vi "get_ecrh_duration.vi"(11 "default":dbl=40.0 format="%#_13g") -> (0 "HTTP status":i32, 1 "ecrh duration":dbl, 2 "time needed to find ECRH duration":i64, 3 "No. Trys":i32, 4 "date/time string":string, 5 "progId":dbl, 6 "last trigger time by codac":i64, 7 "Sucessfull HTTP return?":bool)   [LabVIEW 2014]
uses:
  <vilib>/regexp/Match Regular Expression.xnode
  <vilib>/httpClient/LabVIEWHTTPClient.lvlib
  <vilib>/LVH/i3 JSON/i3-json.lvlib
panel:
  out "is fine?":bool
  out "string length":i32
  out "whole match":string
  out "ECRH substring":string
  out "logbook body":string
  out "after match":string
  out "No. of Trys x > y?":bool
  out "loop status":bool
  out "Tick after":u32 caption="tick after"
  out "tick before":u32
  out "logbook header":string
  out "value":dbl[](array[numeric])
  out "JSON Tree":variant
  out "body":string
  out "headers":string
  out "concatenated string":string
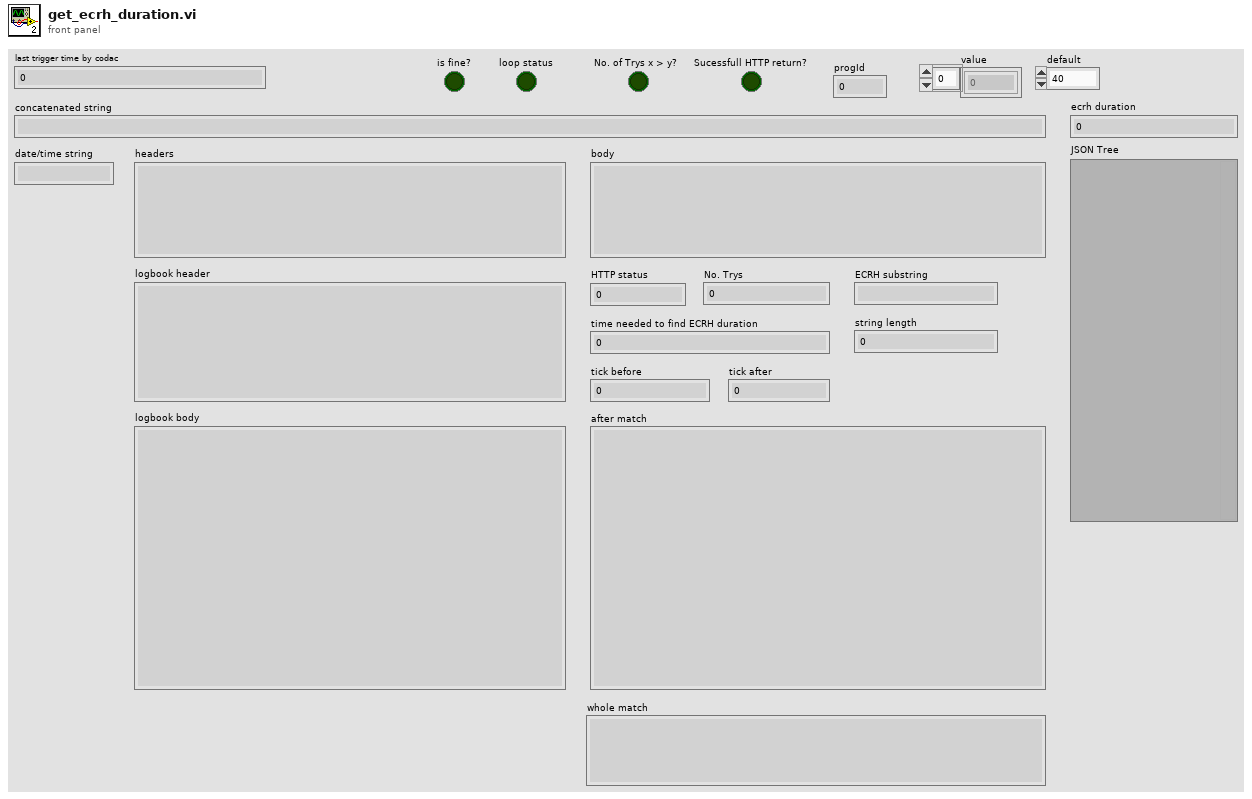
[diagram p1: front panel]
types:
  T1 = typedef "LabVIEWHTTPClient.lvlib/ClientHandle.ctl" = refnum<k1>
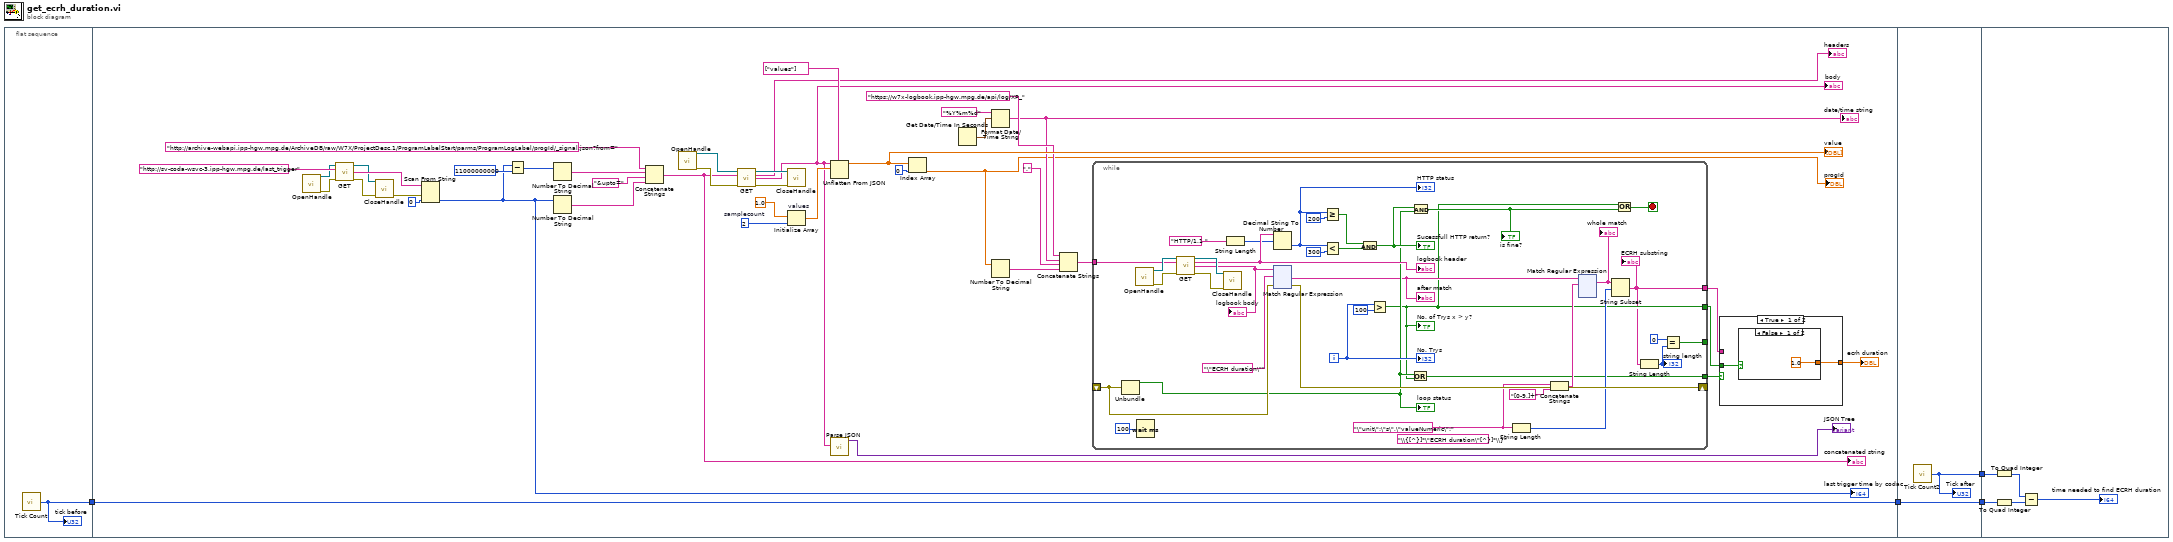
[diagram p0: block diagram]
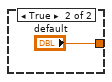
[diagram p2: hidden frame]
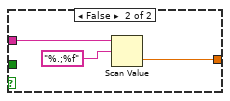
[diagram p3: hidden frame]
diagram:
  n1 = flat-sequence {
    tunnel: [w5] -> w3
    tunnel: [w9] -> w4
    tunnel: w3 -> [w9]
    tunnel: w4 -> [w320]
    tunnel: [w320] -> w2
    tunnel: [w319] -> w1
    tunnel: w2 -> [w324]
    tunnel: w1 -> [w323]
    frame #0 {
      n2 = call "Tick Count"() -> ("Tick Count(mSec)"=w5:u32)
      "tick before" <- w5
    }
    frame #1 {
      w24 = 2  # samplecount
      n3 = call <vilib>:"OpenHandle.vi"() -> ("client handle out"=w43:T1, "error out"=w46:errorcluster)  [unwired: 14 in]
      n4 = call <vilib>:"GET.vi"("client handle"=w43, "url"="http://sv-coda-wsvc-3.ipp-hgw.mpg.de/last_trigger", "error in (no error)"=w46) -> ("client handle out"=w42:T1, "body"=w45:string, "error out"=w41:errorcluster)  [unwired: 9 in, 1 out]
      n5 = call <vilib>:"CloseHandle.vi"("client handle"=w42, "error in (no error)"=w41) -> ("error out"=w40:errorcluster)  [unwired: 13 in]
      n6 = Scan From String(input string=w45, error in=w40, default 1=i64 0 ("default (0 I32)")) -> (output 1=w25:i64)  [unwired: 2 in, 3 out]
      "last trigger time by codac" <- w25
      n7 = Subtract(x=w25, y=i64 11000000000) -> (x-y=w35:i64)
      n8 = Number To Decimal String(number=w35) -> (decimal integer string=w34:string)  [unwired: 1 in]
      n9 = Number To Decimal String(number=w25) -> (decimal integer string=w32:string)  [unwired: 1 in]
      n10 = Concatenate Strings("http://archive-webapi.ipp-hgw.mpg.de/ArchiveDB/raw/W7X/ProjectDesc.1/ProgramLabelStart/parms/ProgramLogLabel/progId/_signal.json?from=", w34, "&upto=", w32) -> (w29:string)
      "concatenated string" <- w29
      n11 = call <vilib>:"OpenHandle.vi"() -> ("client handle out"=w28:T1, "error out"=w31:errorcluster)  [unwired: 14 in]
      n12 = call <vilib>:"GET.vi"("client handle"=w28, "url"=w29, "error in (no error)"=w31) -> ("client handle out"=w27:T1, "headers"=→"headers":string, "body"=w13:string, "error out"=w30:errorcluster)  [unwired: 9 in]
      "body" <- w13
      n13 = call <vilib>:"CloseHandle.vi"("client handle"=w27, "error in (no error)"=w30) -> ()  [unwired: 13 in, 1 out]
      n14 = Initialize Array "values"(1.0 ("element"), w24) -> (w22:dbl[])
      n15 = Unflatten From JSON(path=string[] ["values"], JSON string=w13, type and defaults=w22) -> (value=w21:dbl[])  [unwired: 4 in, 1 out]
      "value" <- w21
      n16 = call <vilib>:"Parse JSON.vi"("JSON String"=w13) -> ("JSON Tree"=→"JSON Tree":variant)  [unwired: 7 in, 3 out]
      n17 = Index Array(array=w21, index=0) -> (element=w16:dbl)
      "progId" <- w16
      n18 = Get Date/Time In Seconds() -> (seconds since 1Jan1904=w39:timestamp)
      n19 = Format Date/Time String(time format string (%c)="%Y%m%d", seconds (now)=w39) -> (date/time string=w18:string)  [unwired: 1 in]
      "date/time string" <- w18
      n20 = Number To Decimal String(number=w16) -> (decimal integer string=w15:string)  [unwired: 1 in]
      n21 = Concatenate Strings("https://w7x-logbook.ipp-hgw.mpg.de/api/log/XP_", w18, "." ("string"), w15) -> (w14:string)
      n22 = while {
        tunnel: w14 -> [w86]
        tunnel: [w60] -> w6
        shift-right: [w70] -> _
        shift-left: _ -> [w69]
        tunnel: [w59] -> w8
        tunnel: [w61] -> w7
        tunnel: [w56] -> _
        i -> [w76]
        stop <- w72 stop-if-true
        (unwired) "\\{[^}]*\"ECRH duration\"[^}]*\\}" ("regular expression")
        w55 = "\"unit\":\"s\",\"valueNumeric\":"
        n23 = Unbundle(w69) -> ("status"=w68:bool)  [unwired: 2 out]
        "loop status" <- w68
        n24 = call <vilib>:"OpenHandle.vi"() -> ("client handle out"=w88:T1, "error out"=w90:errorcluster)  [unwired: 14 in]
        n25 = Wait (ms)(milliseconds to wait=u32 100) -> ()  [unwired: 1 out]
        n26 = call <vilib>:"GET.vi"("client handle"=w88, "url"=w86, "error in (no error)"=w90) -> ("client handle out"=w87:T1, "headers"=w81:string, "body"=w74:string, "error out"=w89:errorcluster)  [unwired: 9 in]
        "logbook header" <- w81
        "logbook body" <- w74
        n27 = call <vilib>:"CloseHandle.vi"("client handle"=w87, "error in (no error)"=w89) -> ()  [unwired: 13 in, 1 out]
        n28 = String Length(string="HTTP/1.1 " ("format string")) -> (length=w79:i32)
        n29 = Decimal String To Number(string=w81, offset=w79) -> (number=w78:i32)  [unwired: 1 in, 1 out]
        "HTTP status" <- w78
        n30 = xnode "Match Regular Expression"("input string"=w74, "regular expression"="\"ECRH duration\"", "error in"=w69) -> ("after match"=w62:string, "error out"=w70:errorcluster)  [unwired: 3 in, 3 out]
        "after match" <- w62
        n31 = Greater Or Equal?(x=w78, y=200) -> (x >= y?=w83:bool)
        n32 = Less?(x=w78, y=300) -> (x < y?=w82:bool)
        n33 = And(x=w83, y=w82) -> (x .and. y?=w71:bool)
        "Sucessfull HTTP return?" <- w71
        n34 = Greater?(x=w76, y=100) -> (0:w61:bool)
        "No. of Trys x > y?" <- w61
        n35 = Or(x=w68, y=w61) -> (x .or. y?=w60:bool)
        n36 = And(x=w71, y=w68) -> (x .and. y?=w73:bool)
        "is fine?" <- w73
        n37 = String Length(string=w55) -> (length=w63:i32)
        n38 = Concatenate Strings(w55, "[0-9.]+") -> (w65:string)
        n39 = xnode "Match Regular Expression"("input string"=w62, "regular expression"=w65) -> ("whole match"=w66:string)  [unwired: 4 in, 4 out]
        "whole match" <- w66
        n40 = String Subset(string=w66, offset (0)=w63) -> (substring=w59:string)  [unwired: 1 in]
        "ECRH substring" <- w59
        n41 = Or(x=w61, y=w73) -> (x .or. y?=w72:bool)
        n42 = String Length(string=w59) -> (length=w58:i32)
        "string length" <- w58
        n43 = Equal?(x=0, y=w58) -> (x = y?=w56:bool)
        "No. Trys" <- w76
      }
      n44 = case shown="True" w6 {
        tunnel: w8 -> [_ w54]
        tunnel: [w49 w52] -> w11
        tunnel: w7 -> [w48 _]
        frame True {
          n45 = case shown="False" w48 {
            tunnel: [1.0 ("default") "default"] -> w49
            frame False {
            }
            frame True {
            }
          }
        }
        frame False {
          n46 = Scan Value(string=w54, format string="%.;%f") -> (value=w52:dbl)  [unwired: 1 in, 1 out]
        }
      }
      "ecrh duration" <- w11
    }
    frame #2 {
      n47 = call "Tick Count2"() -> ("Tick Count(mSec)"=w319:u32)
      "Tick after" <- w319
    }
    frame #3 {
      n48 = To Quad Integer(1:w323) -> (0:w322:i64)
      n49 = To Quad Integer(1:w324) -> (0:w321:i64)
      n50 = Subtract(x=w322, y=w321) -> (x-y=→"time needed to find ECRH duration":i64)
    }
  }
